vi "Table check.vi"(10 "Input table":string[][](array[string])) -> (1 "Incomplete?":bool, 2 "Length":i32)   [LabVIEW 2014]
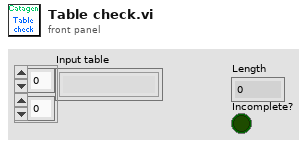
[diagram p1: front panel]
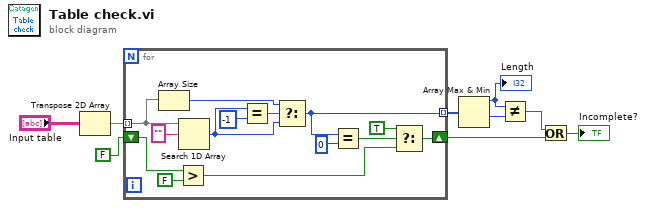
[diagram p0: block diagram]
diagram:
  n1 = Transpose 2D Array(2D array="Input table") -> (transposed array=w9:string[][])
  n2 = for {
    tunnel: w9 -> [w11] mode=indexing
    tunnel: [w10] -> w8 mode=indexing
    shift-right: [w22] -> w3
    shift-left: FALSE -> [w21]
    n3 = Array Size(array=w11) -> (size(s)=w13:i32)
    n4 = Greater?(x=w21, y=FALSE) -> (0:w18:bool)
    n5 = Search 1D Array(1D array=w11, element="") -> (index of element=w12:i32)  [unwired: 1 in]
    n6 = Equal?(x=w12, y=-1) -> (x = y?=w14:bool)
    n7 = Select(t=w13, s=w14, f=w12) -> (s? t:f=w10:i32)
    n8 = Equal?(x=w10, y=0) -> (x = y?=w19:bool)
    n9 = Select(t=TRUE, s=w19, f=w18) -> (s? t:f=w22:bool)
  }
  n10 = Array Max & Min(array=w8) -> (max value=w7:i32, min value=w6:i32)  [unwired: 2 out]
  "Length" <- w7
  n11 = Not Equal?(x=w7, y=w6) -> (x != y?=w4:bool)
  n12 = Or(x=w4, y=w3) -> (x .or. y?=→"Incomplete?":bool)
